vi "Vision Processing.vi"(6 "Std Devs":cluster{"Hue":dbl, "Sat":dbl, "Val":dbl}={"Hue"=4.0, "Sat"=6.0, "Val"=4.0}, 8 "Score Cutoff":dbl(slide)=54.248366013071895 scale=0.0..100.0, 9 "Area Size Limit %":dbl=0.06 format="%#_13g", 10 "Color Components":T4={"Hue"={110.0, 142.0}, "Sat"={138.0, 255.0}, "Val"={139.0, 198.0}} {"Val" scale=0.0..255.0; "Sat" scale=0.0..255.0; "Hue" scale=0.0..255.0 scale format="%#_3g"}, 11 "Image In":T1) -> (0 "Target Info":T3(array[cluster]), 1 "Mask":T1(plugin-control), 3 "Image Out":T1(plugin-control))   [LabVIEW 2013]
uses:
  Program Files (x86)/National Instruments/LabVIEW 2013/examples/FRC/Vision/2014 Target Detection/TargetType.ctl
  <vilib>/vision/Image Controls.llb/IMAQ Image.ctl
panel:
  in  "Tab Control":enum32{"Image Out", "Mask", "Target Info"}(tab)
  in  "Camera Type":enum16{"206", "1011", "1013"}(ring)=enum."1013"
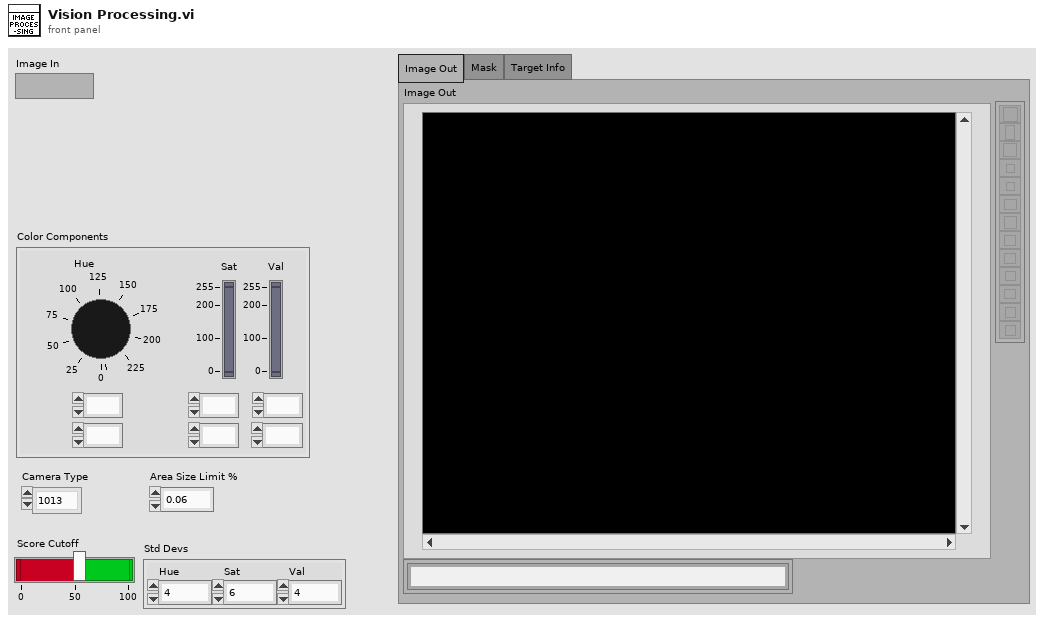
[diagram p1: front panel]
types:
  T1 = typedef "IMAQ Image.ctl" = refnum<image>
  T2 = typedef "TargetType.ctl" = enum16{"Not Hot", "Hot"}
  T3 = cluster{"Scores":cluster{"Total":dbl, "Left":dbl, "Right":dbl, "Ratio":dbl, "Vertical":dbl, "index":i32, "State":T2}, "Verticals":cluster{"Horizontal?":bool, "Aspect Score":dbl, "Rect Score":dbl, cluster{"Left":dbl, "Top":dbl, "Right":dbl, "Bottom":dbl}, "Equiv H":dbl, "Equiv V":dbl}, "Horizontals":cluster{"Horizontal?":bool, "Aspect Score":dbl, "Rect Score":dbl, cluster{"Left":dbl, "Top":dbl, "Right":dbl, "Bottom":dbl}, "Equiv H":dbl, "Equiv V":dbl}, "Distance ft":dbl, "Center":cluster{"X":dbl, "Y":dbl}}[]
  T4 = cluster{"Hue":cluster{dbl, dbl}, "Sat":cluster{dbl, dbl}, "Val":cluster{dbl, dbl}}
  T5 = cluster{"Horizontal":bool, "Aspect Score":dbl, "Rect Score":dbl, cluster{"Left":dbl, "Top":dbl, "Right":dbl, "Bottom":dbl}, "Equiv H":dbl, "Equiv V":dbl}[]
  T6 = cluster{cluster{dbl, dbl}, cluster{dbl, dbl}, cluster{dbl, dbl}}
  T7 = cluster{"Scores":cluster{"Total":dbl, "Left":dbl, "Right":dbl, "Ratio":dbl, "Vertical":dbl, "index":i32, "State":T2}, "Verticals":cluster{"Horizontal?":bool, "Aspect Score":dbl, "Rect Score":dbl, cluster{"Left":dbl, "Top":dbl, "Right":dbl, "Bottom":dbl}, "Equiv H":dbl, "Equiv V":dbl}, "Horizontals":cluster{"Horizontal?":bool, "Aspect Score":dbl, "Rect Score":dbl, cluster{"Left":dbl, "Top":dbl, "Right":dbl, "Bottom":dbl}, "Equiv H":dbl, "Equiv V":dbl}, "Validated":bool}[]
  T8 = cluster{"Scores":cluster{"Total":dbl, "Left":dbl, "Right":dbl, "Ratio":dbl, "Vertical":dbl, "index":i32, "State":T2}, "Verticals":cluster{"Horizontal?":bool, "Aspect Score":dbl, "Rect Score":dbl, cluster{"Left":dbl, "Top":dbl, "Right":dbl, "Bottom":dbl}, "Equiv H":dbl, "Equiv V":dbl}, "Horizontals":cluster{"Horizontal?":bool, "Aspect Score":dbl, "Rect Score":dbl, cluster{"Left":dbl, "Top":dbl, "Right":dbl, "Bottom":dbl}, "Equiv H":dbl, "Equiv V":dbl}, "Distance (ft)":dbl, "Target Center (-1 to 1)":cluster{"X":dbl, "Y":dbl}}[]
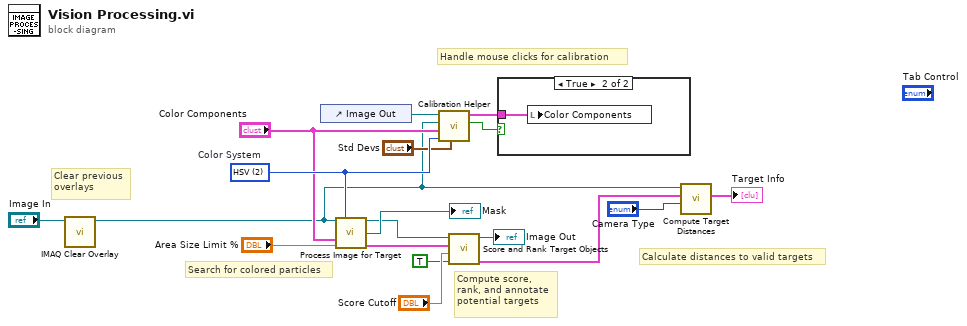
[diagram p0: block diagram]
diagram:
  w8 = u16 2 items=["RGB", "HSL", "HSV", "HSI"]  # Color System
  # "Clear previous\noverlays"
  # "Calculate distances to valid targets"
  # "Search for colored particles"
  # "Handle mouse clicks for calibration"
  # "Compute score,\nrank, and annotate\npotential targets"
  n1 = call "IMAQ Clear Overlay"("Image"="Image In") -> ("Image Out"=w3:T1)  [unwired: 9 in, 1 out]
  n2 = control-ref of="Image Out"() -> (w9:refnum<vi>)
  n3 = call "Process Image for Target.vi"("Src Image"=w3, "Color Mode"=w8, "Color Components"="Color Components", "Area Cutoff %"="Area Size Limit %") -> ("Src Image Out"=w16:T1, "Threshold"=→"Mask":T1, "Particles"=w13:T5)  [unwired: 9 in]
  n4 = call "Calibration Helper.vi"("Std Devs"="Std Devs", "Color Mode"=w8, "Color Components"="Color Components", "Image"=w3, "Image Ctl Refnum"=w9) -> ("Changed"=w4:bool, "output color"=w6:T6)  [unwired: 5 in]
  n5 = call "Score and Rank Target Objects.vi"("Annotate"=TRUE, "Score Limit"="Score Cutoff", "Particles"=w13, "Image in"=w16) -> ("Target Info"=w12:T7, "Annotated Image"=→"Image Out":T1)  [unwired: 6 in]
  n6 = case shown="True" w4 {
    tunnel: w6 -> [_ w19]
    frame False {
    }
    frame True {
      n7 = local write "Color Components"(w19) -> ()
    }
  }
  n8 = call "Compute Target Distances.vi"("Camera Type"="Camera Type", "Target Info"=w12, "Image in"=w3) -> ("Target Info"=→"Target Info":T8)  [unwired: 6 in, 2 out]
